vi "DAQ_Close.vi"(1 "error in":errorcluster, 2 "task in":refnum<k21>) -> (0 "error out":errorcluster)   [LabVIEW 2024]
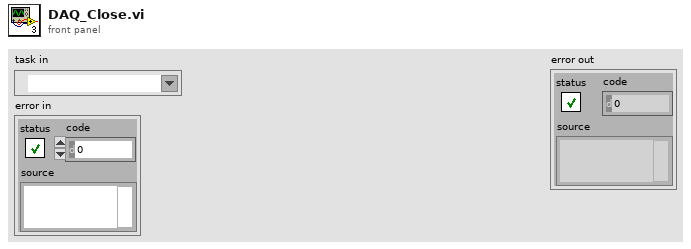
[diagram p1: front panel]
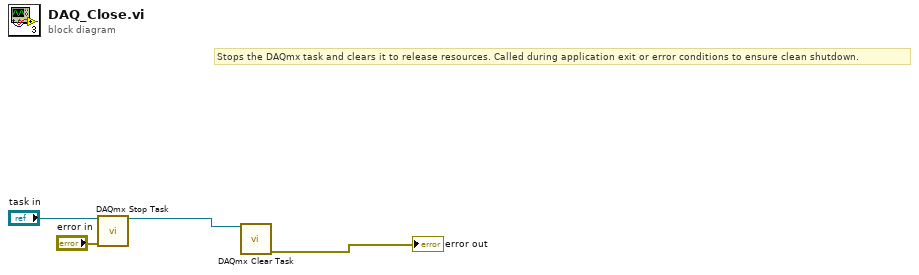
[diagram p0: block diagram]
diagram:
  # "Stops the DAQmx task and clears it to release resources. Called during application exit or error conditions to ensure clean shutdown."
  n1 = call <vilib>:"DAQmx Stop Task.vi"("task/channels in"="task in", "error in"="error in") -> ("task out"=w1:refnum<k21>)  [unwired: 12 in, 1 out]
  n2 = call <vilib>:"DAQmx Clear Task.vi"("task in"=w1) -> ("error out"=→"error out":errorcluster)  [unwired: 14 in]
